vi "Init HTTP Server.vi"(8 "error in (no error)":errorcluster, 11 "SOL-Server in":refnum<class "SOL-Server.lvclass">) -> (0 "error out":errorcluster, 3 "SOL-Server out":refnum<class "SOL-Server.lvclass">)   [LabVIEW 2020, in "Summer of LabVIEW.lvlib" / "SOL-Server.lvclass"]
uses:
  SOL-Server.lvclass
  <vilib>/IlluminatedG/IG HTTP Server/HTTP Server/Server Caching.ctl
  <vilib>/IlluminatedG/IG HTTP Server/HTTP Server/HTTPS Options.ctl
  SOL-Server.lvclass/SOL-Server.ctl
  <vilib>/IlluminatedG/IG HTTP Server/HTTP Server/StandardFileServe/StandardFileServe.lvclass
  C:/Program Files (x86)/National Instruments/LabVIEW 2020/vi.lib/IlluminatedG/IG HTTP Server/HTTP Server/Handler/Handler.lvclass
  <vilib>/IlluminatedG/IG HTTP Server/HTTP Server/Server/Add Connection Handler.vi
  <vilib>/IlluminatedG/IG HTTP Server/HTTP Server/Server/Add Request Handler.vi
  <vilib>/IlluminatedG/IG HTTP Server/HTTP Server/Server/Add Route Handler.vi
  <vilib>/IlluminatedG/IG HTTP Server/HTTP Server/Server/Add Controller Handler.vi
  <vilib>/IlluminatedG/IG HTTP Server/HTTP Server/Server/Add Controller.vi
  <vilib>/IlluminatedG/IG HTTP Server/HTTP Server/Server/Add Response Handler.vi
  <vilib>/IlluminatedG/IG HTTP Server/HTTP Server/Server/Add Complete Handler.vi
  <vilib>/IlluminatedG/IG HTTP Server/HTTP Server/Server/Add Exception Handler.vi
  <vilib>/IlluminatedG/IG HTTP Server/HTTP Server/Connection Handler/Connection Handler.lvclass
  <vilib>/IlluminatedG/IG HTTP Server/HTTP Server/Request Handler/Request Handler.lvclass
  <vilib>/IlluminatedG/IG HTTP Server/HTTP Server/Route Handler/Route Handler.lvclass
  <vilib>/IlluminatedG/IG HTTP Server/HTTP Server/Controller Handler/Controller Handler.lvclass
  <vilib>/IlluminatedG/IG HTTP Server/HTTP Server/Controller/Controller.lvclass
  <vilib>/IlluminatedG/IG HTTP Server/HTTP Server/Response Handler/Response Handler.lvclass
  <vilib>/IlluminatedG/IG HTTP Server/HTTP Server/Complete Handler/Complete Handler.lvclass
  <vilib>/IlluminatedG/IG HTTP Server/HTTP Server/Exception Handler/Exception Handler.lvclass
  <vilib>/IlluminatedG/IG HTTP Server/HTTP Server/Handler/Handler.lvclass
  <vilib>/IlluminatedG/IG HTTP Server/HTTP Server/Server/Server.lvclass
  <vilib>/IlluminatedG/IG HTTP Server/HTTP Server/Session/Session.lvclass
  <vilib>/IlluminatedG/IG HTTP Server/HTTP Server/HTTP Server.lvlib
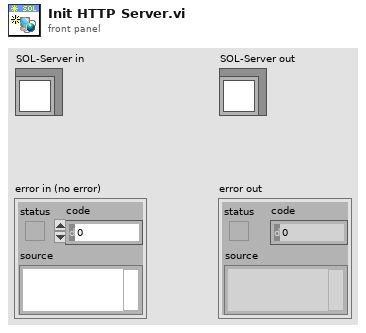
[diagram p1: front panel]
types:
  T1 = typedef "HTTP Server.lvlib/HTTPS Options.ctl" = cluster{"HTTPS Enabled":bool, "Private Key":path, "Private Key Format":enum32{"PKCS#8 (PEM)", "PKCS#8 (DER)"}, "Public Cert":path, "Public Cert Format":enum32{"X.509 (PEM)"}, "Always Secure?":bool, "HTTPS Port (443)":u16}
  T2 = typedef "HTTP Server.lvlib/Server Caching.ctl" = cluster{"Auto Cache Static Files":bool, "Cache Folder":path, "Memory Caching Bytes Limit":i32, "Memory Caching Age Limit":dbl, "File Caching Age Limit":dbl, "Default Cache Max Age":i32}
  T3 = typedef "Summer of LabVIEW.lvlib/SOL-Server.lvclass/Paths.ctl" = cluster{"Web Root":path, "Sessions":path, "Config":path, "SQLite DB File":path, "SSL Cert Folder":path}
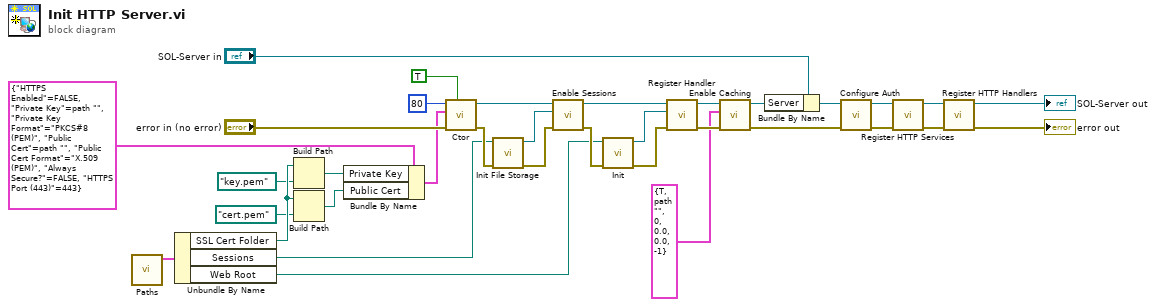
[diagram p0: block diagram]
diagram:
  n1 = call "Paths.vi"() -> ("Paths"=w29:T3)  [unwired: 11 in]
  n2 = Unbundle By Name(w29) -> ("SSL Cert Folder"=w9:path, "Sessions"=w5:path, "Web Root"=w4:path)
  n3 = Build Path(base path=w9, name or relative path=path "key.pem") -> (appended path=w2:path)
  n4 = Build Path(base path=w9, name or relative path=path "cert.pem") -> (appended path=w1:path)
  n5 = Bundle By Name(cluster=T1 {"HTTPS Enabled"=FALSE, "Private Key"=path "", "Private Key Format"=enum."PKCS#8 (PEM)", "Public Cert"=path "", "Public Cert Format"=enum."X.509 (PEM)", "Always Secure?"=FALSE, "HTTPS Port (443)"=443} ("HTTPS Options (Disabled)"), "Private Key"=w2, "Public Cert"=w1) -> (w3:T1)
  n6 = call <vilib>:"Ctor.vi"("Debug (F)"=TRUE, "error in (no error)"="error in (no error)", "HTTPS Options (Disabled)"=w3, "HTTP Port (80)"=u16 80 ("Port (8080)")) -> ("error out"=w33:errorcluster, "Server out"=w28:refnum<class "Server.lvclass">)  [unwired: 6 in]
  n7 = call <vilib>:"Init File Storage.vi"("error in (no error)"=w33, "Session Storage Folder"=w5) -> ("error out"=w26:errorcluster, "Session out"=w27:refnum<class "Session.lvclass">)  [unwired: 8 in]
  n8 = call <vilib>:"Enable Sessions.vi"("error in (no error)"=w26, "Session Implementation"=w27, "Server in"=w28) -> ("error out"=w34:errorcluster, "Server out"=w25:refnum<class "Server.lvclass">)  [unwired: 7 in]
  n9 = call <vilib>:"Init.vi"("error in (no error)"=w34, "Public Root"=w4) -> ("error out"=w23:errorcluster, "StandardFileServe out"=w24:refnum<class "StandardFileServe.lvclass">)  [unwired: 8 in]
  n10 = call <vilib>:"Register Handler.vi"("error in (no error)"=w23, "Handler"=w24, "Server in"=w25) -> ("error out"=w13:errorcluster, "Server out"=w14:refnum<class "Server.lvclass">)  [unwired: 7 in]
  n11 = call <vilib>:"Enable Caching.vi"("error in (no error)"=w13, "Server Caching"=T2 {"Auto Cache Static Files"=TRUE, "Cache Folder"=path "", "Memory Caching Bytes Limit"=0, "Memory Caching Age Limit"=0.0, "File Caching Age Limit"=0.0, "Default Cache Max Age"=-1}, "Server in"=w14) -> ("error out"=w11:errorcluster, "Server out"=w12:refnum<class "Server.lvclass">)  [unwired: 7 in]
  n12 = Bundle By Name(cluster="SOL-Server in", "Server"=w12) -> (w17:refnum<class "SOL-Server.lvclass">)
  n13 = call "Configure Auth.vi"("error in (no error)"=w11, "SOL-Server in"=w17) -> ("error out"=w15:errorcluster, "SOL-Server out"=w16:refnum<class "SOL-Server.lvclass">)  [unwired: 8 in]
  n14 = call "Register HTTP Services.vi"("error in (no error)"=w15, "SOL-Server in"=w16) -> ("error out"=w20:errorcluster, "SOL-Server out"=w21:refnum<class "SOL-Server.lvclass">)  [unwired: 8 in]
  n15 = call "Register HTTP Handlers.vi"("error in (no error)"=w20, "SOL-Server in"=w21) -> ("error out"=→"error out":errorcluster, "SOL-Server out"=→"SOL-Server out":refnum<class "SOL-Server.lvclass">)  [unwired: 8 in]
